vi "SLSC_Get_Properties.vi"(6 "SLSC Dynamic Inputs":T1[](array[typedef]), 7 "LoopDuration(ms)":u32, 8 "error in":errorcluster, 10 "session in":refnum<k21>, 11 "SLSC Module Name":refnum<k21>) -> (0 "error out":errorcluster, 1 "Values":dbl[](array[numeric]), 2 "session out":refnum<k21>, 3 "SLSC Module Name":refnum<k21>)   [LabVIEW 2015, in "SLSC-12201 DIO Engine.lvlib"]
uses:
  SLSC-12201 DIO Engine.lvlib
  Shared/SLSC Dynamic Channel.ctl
  Shared/SLSC Dynamic Channel Type.ctl
  <vilib>/SLSC/Get Generic Property (U64).vi
  <vilib>/SLSC/Get Generic Property (U32).vi
  <vilib>/SLSC/Get Generic Property (String).vi
  <vilib>/SLSC/Get Generic Property (I64).vi
  <vilib>/SLSC/Get Generic Property (I32).vi
  <vilib>/SLSC/Get Generic Property (DBL).vi
  <vilib>/SLSC/Get Generic Property (Bool).vi
  <vilib>/SLSC/SLSC.lvlib
  Shared/SLSC-12201 DIO Shared.lvlib
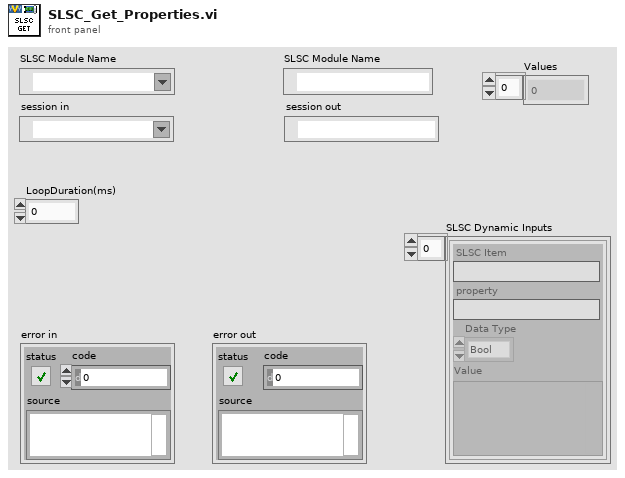
[diagram p1: front panel]
types:
  T1 = typedef "SLSC-12201 DIO Shared.lvlib/SLSC Dynamic Channel.ctl" = cluster{"SLSC Item":string, "property":string, "Data Type":T2, "Value":variant}
  T2 = typedef "SLSC-12201 DIO Shared.lvlib/SLSC Dynamic Channel Type.ctl" = enum16{"Bool", "Double", "I32", "I64", "String", "U32", "U64", "EnumI32"}
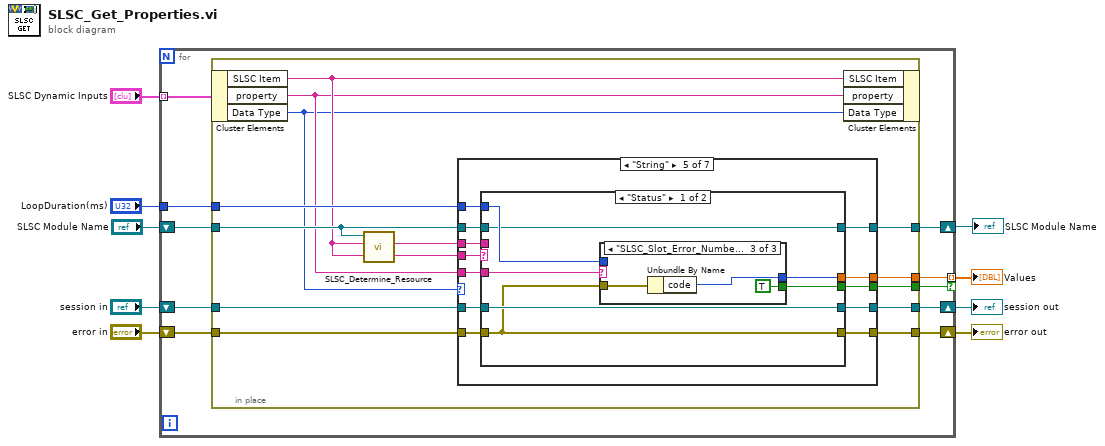
[diagram p0: block diagram]
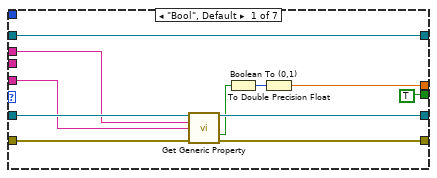
[diagram p2: hidden frame]
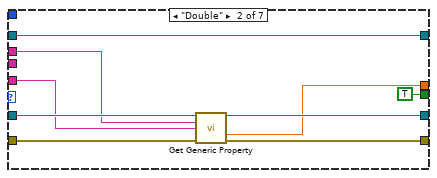
[diagram p3: hidden frame]
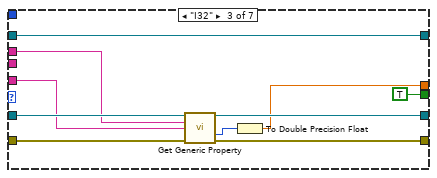
[diagram p4: hidden frame]
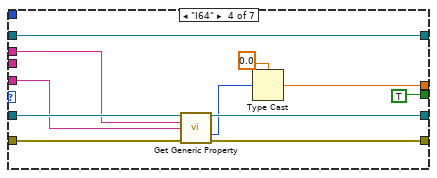
[diagram p5: hidden frame]
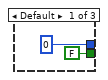
[diagram p6: hidden frame]
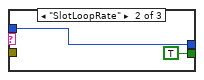
[diagram p7: hidden frame]
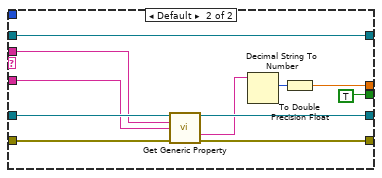
[diagram p8: hidden frame]
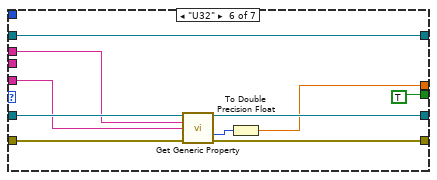
[diagram p9: hidden frame]
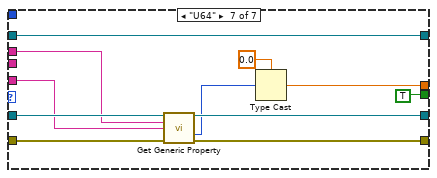
[diagram p10: hidden frame]
diagram:
  n1 = for {
    tunnel: "SLSC Dynamic Inputs" -> [w10] mode=indexing
    shift-right: [w16] -> w6
    shift-left: "session in" -> [w19]
    shift-right: [w14] -> w3
    shift-left: "SLSC Module Name" -> [w11]
    shift-right: [w15] -> w9
    shift-left: "error in" -> [w18]
    tunnel: [w17] -> w2 mode=indexing if=w13
    tunnel: "LoopDuration(ms)" -> [w12]
    n2 = in-place {
      in-place-border: w19 -> [w32]
      in-place-border: w18 -> [w31]
      in-place-border: [w30] -> w17
      in-place-border: [w29] -> w16
      in-place-border: [w28] -> w15
      in-place-border: [w27] -> w14
      in-place-border: [w26] -> w13
      in-place-border: w12 -> [w25]
      in-place-border: w11 -> [w24]
      n3 = in-place-cluster #1(w10) -> ("SLSC Item"=w22:string, "property"=w21:string, "Data Type"=w20:T2)
      n4 = call "SLSC_Determine_Resource.vi"("SLSC Item"=w22, "SLSC Module Name"=w24) -> ("Resource"=w23:string)  [unwired: 9 in]
      n5 = case shown="\"String\"" w20 {
        tunnel: w32 -> [w43 w52 w62 w73 w85 w120 w131]
        tunnel: [w42 w51 w61 w72 w84 w119 w130] -> w29
        tunnel: w21 -> [w41 w50 w60 w71 w83 w118 w129]
        tunnel: w22 -> [_ _ _ _ w79 _ _]
        tunnel: w24 -> [w40 w49 w59 w70 w77 w117 w128]
        tunnel: [w40 w49 w59 w70 w75 w117 w128] -> w27
        tunnel: w31 -> [w39 w48 w58 w69 w82 w116 w127]
        tunnel: [w38 w47 w57 w68 w81 w115 w126] -> w28
        tunnel: [w35 w46 w56 w67 w80 w114 w125] -> w30
        tunnel: [TRUE TRUE TRUE TRUE w78 TRUE TRUE] -> w26
        tunnel: w25 -> [_ _ _ _ w76 _ _]
        tunnel: w23 -> [w33 w44 w53 w63 w74 w111 w121]
        frame "Bool", Default {
          n6 = call-poly <vilib>:"Get Generic Property.vi"("session in"=w43, "resources"=w33, "property"=w41, "error in (no error)"=w39) -> ("session out"=w42:refnum<k21>, "property value"=w37:bool, "error out"=w38:errorcluster)  [unwired: 9 in]
          n7 = Boolean To (0,1)(Boolean=w37) -> (0, 1=w36:i16)
          n8 = To Double Precision Float(number=w36) -> (double precision float=w35:dbl)
        }
        frame "Double" {
          n9 = call-poly <vilib>:"Get Generic Property.vi"("session in"=w52, "resources"=w44, "property"=w50, "error in (no error)"=w48) -> ("session out"=w51:refnum<k21>, "property value"=w46:dbl, "error out"=w47:errorcluster)  [unwired: 9 in]
        }
        frame "I32" {
          n10 = call-poly <vilib>:"Get Generic Property.vi"("session in"=w62, "resources"=w53, "property"=w60, "error in (no error)"=w58) -> ("session out"=w61:refnum<k21>, "property value"=w55:i32, "error out"=w57:errorcluster)  [unwired: 9 in]
          n11 = To Double Precision Float(number=w55) -> (double precision float=w56:dbl)
        }
        frame "I64" {
          n12 = call-poly <vilib>:"Get Generic Property.vi"("session in"=w73, "resources"=w63, "property"=w71, "error in (no error)"=w69) -> ("session out"=w72:refnum<k21>, "property value"=w66:i64, "error out"=w68:errorcluster)  [unwired: 9 in]
          n13 = Type Cast(type=0.0, x=w66) -> (*(type *) &x=w67:dbl)
        }
        frame "String" {
          n14 = case shown="\"Status\"" w79 {
            tunnel: w85 -> [w92 w110]
            tunnel: [w92 w109] -> w84
            tunnel: w83 -> [w87 w108]
            tunnel: w77 -> [w86 w101]
            tunnel: w82 -> [w88 w107]
            tunnel: [w88 w106] -> w81
            tunnel: [w91 w105] -> w80
            tunnel: [w89 TRUE] -> w78
            tunnel: w76 -> [w90 _]
            tunnel: [w86 w101] -> w75
            tunnel: w74 -> [_ w100]
            frame "Status" {
              n15 = case shown="\"SLSC_Slot_Error_Number\"" w87 {
                tunnel: [u32 0 ("LoopDuration(ms)") w95 w97] -> w91
                tunnel: w90 -> [_ w95 _]
                tunnel: [FALSE TRUE TRUE] -> w89
                tunnel: w88 -> [_ _ w98]
                frame Default {
                }
                frame "SlotLoopRate" {
                }
                frame "SLSC_Slot_Error_Number" {
                  n16 = Unbundle By Name(w98) -> ("code"=w97:i32)
                }
              }
            }
            frame Default {
              n17 = call-poly <vilib>:"Get Generic Property.vi"("session in"=w110, "resources"=w100, "property"=w108, "error in (no error)"=w107) -> ("session out"=w109:refnum<k21>, "property value"=w104:string, "error out"=w106:errorcluster)  [unwired: 9 in]
              n18 = Decimal String To Number(string=w104) -> (number=w103:i32)  [unwired: 2 in, 1 out]
              n19 = To Double Precision Float(number=w103) -> (double precision float=w105:dbl)
            }
          }
        }
        frame "U32" {
          n20 = call-poly <vilib>:"Get Generic Property.vi"("session in"=w120, "resources"=w111, "property"=w118, "error in (no error)"=w116) -> ("session out"=w119:refnum<k21>, "property value"=w113:u32, "error out"=w115:errorcluster)  [unwired: 9 in]
          n21 = To Double Precision Float(number=w113) -> (double precision float=w114:dbl)
        }
        frame "U64" {
          n22 = call-poly <vilib>:"Get Generic Property.vi"("session in"=w131, "resources"=w121, "property"=w129, "error in (no error)"=w127) -> ("session out"=w130:refnum<k21>, "property value"=w124:u64, "error out"=w126:errorcluster)  [unwired: 9 in]
          n23 = Type Cast(type=0.0, x=w124) -> (*(type *) &x=w125:dbl)
        }
      }
      n24 = in-place-cluster #1("SLSC Item"=w22, "property"=w21, "Data Type"=w20) -> ()  [unwired: 1 out]
    }
  }
  "error out" <- w9
  "Values" <- w2
  "session out" <- w6
  "SLSC Module Name" <- w3
